vi "PicoScope4000SetDataBufferWithMode.vi"(5 "enabled array":i16[](array[numeric]), 7 "Buffer and Transfer Settings":T2 {"Down-Sample Mode" items=["RAW none", "None", "Aggregate", "Decimate", "Average"]; "Down Sample Ratio" step=1; "Samples" format="%_6p"}, 8 "error in (no error)":errorcluster, 10 "Data Pointers In":T1, 11 "handle in":i16) -> (0 "error out":errorcluster, 3 "handle out":i16)   [LabVIEW 2009]
doc: "Calls SetDataBuffers, and assigns Pico buffers"
uses:
  ps4000.dll
  shared/PicoBuffers.ctl
  shared/Buffer and Transfer Settings.ctl
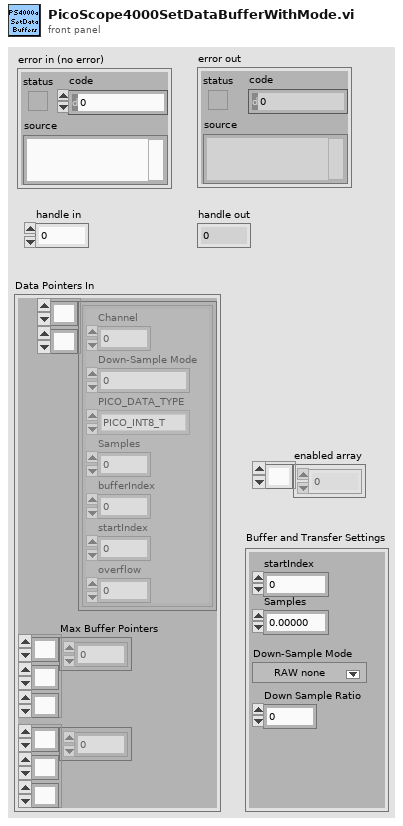
[diagram p1: front panel]
types:
  T1 = typedef "PicoBuffers.ctl" = cluster{"Max Buffer Pointers":u64[][][], "Min Buffer Pointers":u64[][][], "StreamingDataInfo":cluster{"Channel":u32, "Down-Sample Mode":u32, "PICO_DATA_TYPE":enum32{"PICO_INT8_T", "PICO_INT16_T", "PICO_INT32_T", "PICO_UINT32_T", "PICO_INT64_T", ""}, "Samples":i32, "bufferIndex":u64, "startIndex":i32, "overflow":i16}[][]}
  T2 = typedef "Buffer and Transfer Settings.ctl" = cluster{"startIndex":u64, "Samples":u64, "Down Sample Ratio":u64, "Down-Sample Mode":u32}
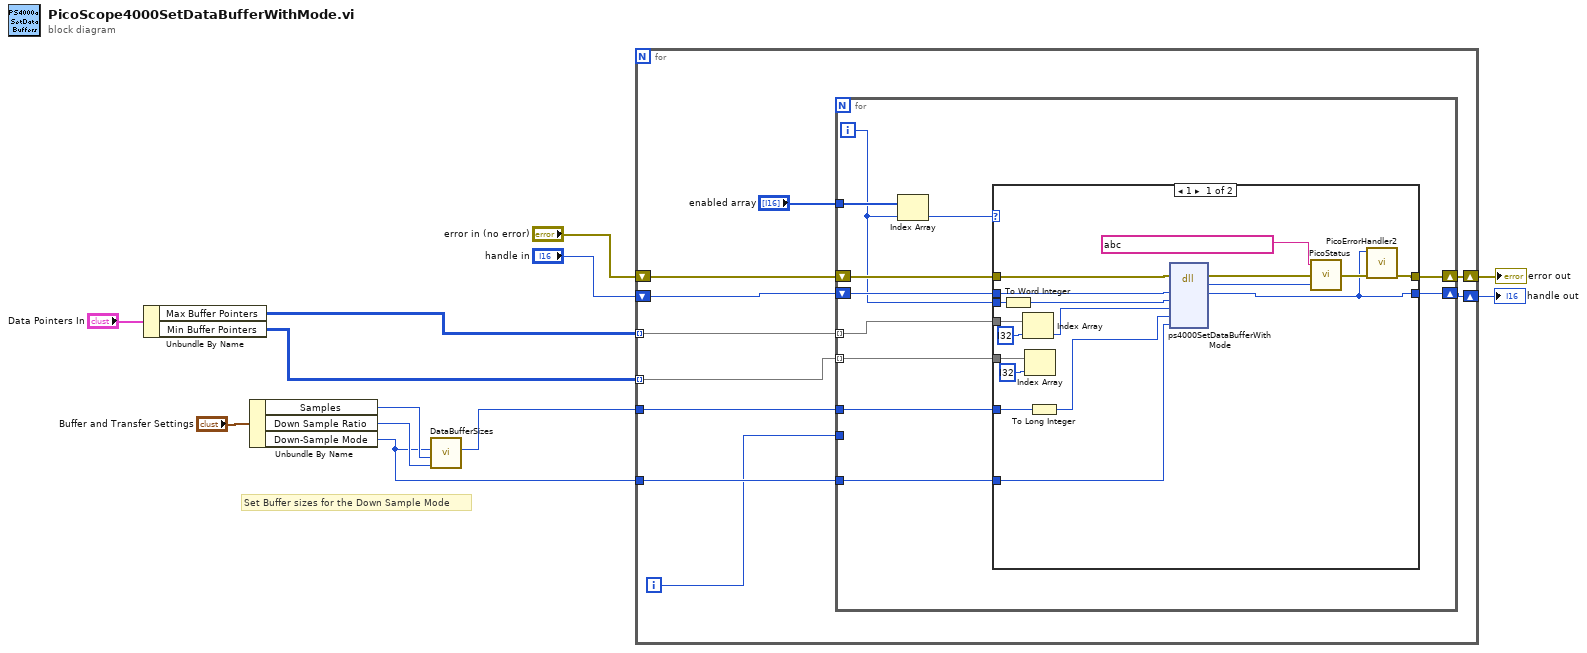
[diagram p0: block diagram]
diagram:
  # "Set Buffer sizes for the Down Sample Mode"
  n1 = Unbundle By Name("Data Pointers In") -> ("Max Buffer Pointers"=w2:u64[][][], "Min Buffer Pointers"=w1:u64[][][])
  n2 = Unbundle By Name("Buffer and Transfer Settings") -> ("Samples"=w4:u64, "Down Sample Ratio"=w5:u64, "Down-Sample Mode"=w3:u32)
  n3 = call "DataBufferSizes.vi"("Down Sample Ratio"=w5, "Number of Samples"=w4, "Down-Sample Mode"=w3) -> ("Max Buffer Size"=w6:i32)  [unwired: 7 in, 1 out]
  n4 = for {
    tunnel: w6 -> [w18]
    tunnel: w3 -> [w17]
    tunnel: w2 -> [w16] mode=indexing
    tunnel: w1 -> [w15] mode=indexing
    shift-right: [w22] -> w11
    shift-left: "error in (no error)" -> [w20]
    shift-right: [w21] -> w10
    shift-left: "handle in" -> [w19]
    i -> [w13]
    n5 = for {
      tunnel: w17 -> [w33]
      tunnel: w18 -> [w28]
      tunnel: "enabled array" -> [w30]
      tunnel: w16 -> [w27] mode=indexing
      shift-right: [w26] -> w22
      shift-left: w20 -> [w32]
      tunnel: w15 -> [w25] mode=indexing
      shift-right: [w24] -> w21
      shift-left: w19 -> [w31]
      tunnel: w13 -> [_]
      i -> [w23]
      n6 = Index Array(array=w30, index=w23) -> (element=w29:i16)
      n7 = case shown="1" w29 {
        tunnel: w23 -> [w48 _]
        tunnel: w32 -> [w43 w53]
        tunnel: w31 -> [w42 w52]
        tunnel: w33 -> [w34 _]
        tunnel: [w50 w53] -> w26
        tunnel: [w35 w52] -> w24
        tunnel: w28 -> [w49 _]
        tunnel: w27 -> [w46 _]
        tunnel: w25 -> [w44 _]
        frame #0 {
          n8 = To Word Integer(number=w48) -> (16bit integer=w41:i16)
          n9 = Index Array(array=w46, index=i32 ?) -> (element=w40:u64)
          n10 = Index Array(array=w44, index=i32 ?) -> ()  [unwired: 1 out]
          n11 = To Long Integer(number=w49) -> (32bit integer=w39:i32)
          n12 = dll-call lib="ps4000.dll" fn="ps4000SetDataBufferWithMode" ("ps3000.dll:_ps3000_open_unit@0")(error in=w43, "handle"=w42, "channel"=w41, "bufferMax"=w40, "bufferLth"=w39, "mode"=w34) -> (error out=w38:errorcluster, "PICO_STATUS"=w36:u32, "handle"=w35:i16)  [unwired: 6 in, 1 out]
          n13 = call "PicoStatus.vi"("PICO STATUS"=w36, "error in"=w38, "source"=string ?) -> ("error out"=w37:errorcluster)
          n14 = call "PicoErrorHandler2.vi"("error in (no error)"=w37, "handle In"=w35) -> ("error out"=w50:errorcluster)  [unwired: 9 in]
        }
        frame #1 {
        }
      }
    }
  }
  "error out" <- w11
  "handle out" <- w10
